vi "GA_Search_Main_Function.vi"(6 "ReInitialize?":bool, 8 "Stop ButtonRef in":refnum<vi>, 9 "Accuracies Listbox Ref in":refnum<vi>, 10 "Fitness Chart Ref in":refnum<vi>, 11 "GA Metaparameters in":T1={"Training Data Path"=path "", "Test Data Path"=path "", "True Labels for Test Trials"=path "", "ClassifierType"=enum."Multilayer perceptron", "SVM Options"={"Kernel"=enum."Linear", "Degree"=0, "Gamma"=0.0, "Coefficient"=0.0, "Sigma"=0.0, "Cache(MB)"=0.0}, "GA Parameters"={"Population size"=0, "Generations no."=0, "Crossover probabality"=0.0, "Mutation mode"=enum."one-point, fixed rate", "Creep mutation"=FALSE, "Mutation rate"=0.0, "Min mutation rate"=0.0, "Max mutation rate"=0.0, "Relative fitness differential"=0.0, "Reproduction plan"=enum."Full generational replacement", "Elitism"=FALSE, "FeaturesPerChannel"=0}, "Use equal number of trials?"=FALSE, "Classifier Metaparameter"=5.0, "ClassifierQualityMeasure"=enum."Accuracy"} {"Classifier Metaparameter" min=0.0 max=100.0 step=0.1 format="%#_2g"; "GA Parameters"."Relative fitness differential" min=0.0 max=1.0; "GA Parameters"."Max mutation rate" min=0.0 max=1.0; "GA Parameters"."Min mutation rate" min=0.0 max=1.0; "GA Parameters"."Mutation rate" min=0.0 max=1.0; "GA Parameters"."Crossover probabality" min=0.0 max=1.0; "GA Parameters"."Generations no." min=1; "GA Parameters"."Population size" min=1}) -> (0 "Accuracies out (double)":dbl[](array[numeric]), 3 "Accuracies out (string)":string[](array[string]))   [LabVIEW 2016, in "GA.lvlib"]
uses:
  _vlib/GA_tSolution progress.ctl
  _vlib/GA_tPopulation.ctl
  _vlib/GA_metaParameters.ctl
  4. Accuracy Assessment for EEG Classification/_vlib/CU_ClassifierTypes.ctl
  <vilib>/vision/Classification.llb/IMAQ SVM Kernel Options.ctl
  _vlib/GA_tParameters.ctl
  4. Accuracy Assessment for EEG Classification/_vlib/CU_ClassifierQualityMeasure.ctl
  _vlib/GA_ApplicationState.ctl
  4. Accuracy Assessment for EEG Classification/_vlib/ClassifierClass.lvclass
  4. Accuracy Assessment for EEG Classification/_vlib/ClassifierClass.lvclass/ClassifierClass.ctl
  _vlib/GA_tFitness Function.ctl
  _vlib/GA.lvlib
  4. Accuracy Assessment for EEG Classification/Classifier.lvlib
panel:
  out "Number of classes":i32 caption="Число классов"
  out "Feature Vector Length":i32 caption="Длина вектора признаков"
  out "Number of True Labels":i32 caption="Число меток классов"
  out "Number of Test Trials":i32 caption="Число тестовых проб"
  out "Number of Training Trials":i32 caption="Число обучающих проб"
  out "Number of trials of each class":i32[](array[numeric]) caption="Число проб каждого класса"
  out "Population Notifier":refnum<notifier>
  out "Solution Notifier":refnum<notifier>
  out "Application State":string caption="Состояние"
  # "This VI is a part of BCI Design library, http://www.ru-bci.org \nCopyright © 2020, Sotnikov Peter, All rights reserved. License: GNU GPLv3"
  # "Поколение"
  # "Точность\nна тестовой\nвыборке"
  # "Размерность\nвектора\nпризнаков"
  # "Точность\nна обучающей\nвыборке"
  # "Точность\nна контрол. \nвыборке"
  # "Результаты чтения данных"
  # "Размер популяции"
  # "Число поколений"
  # "Вероятность скрещивания (кроссовера)"
  # "Тип мутации"
  # "Вероятность мутации"
  # "Минимальная вероятность мутации"
  # "Максимальная вероятность мутации"
  # "Способ включения потомков в популяцию"
  # "Использовать элитизм?"
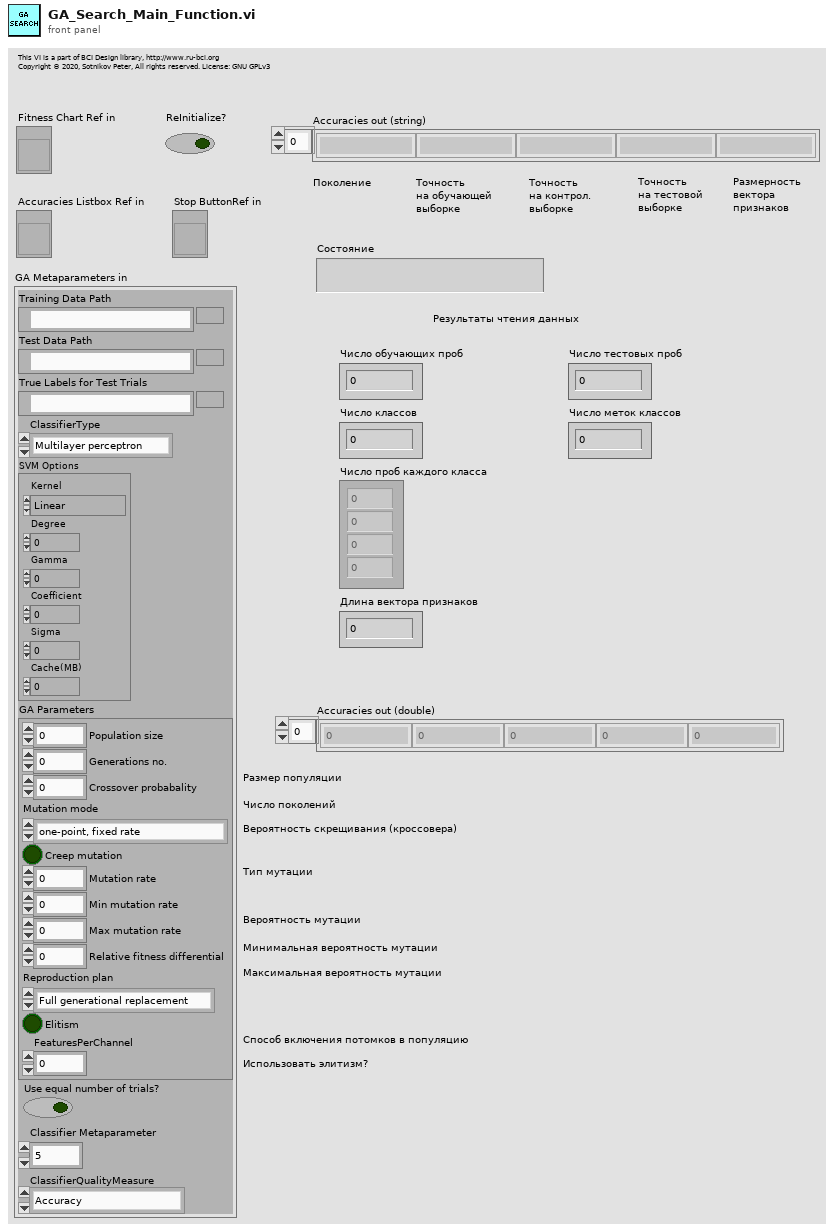
[diagram p1: front panel]
types:
  T1 = typedef "GA.lvlib/GA_metaParameters.ctl" = cluster{"Training Data Path":path, "Test Data Path":path, "True Labels for Test Trials":path, "ClassifierType":T2, "SVM Options":T3, "GA Parameters":T4, "Use equal number of trials?":bool, "Classifier Metaparameter":dbl, "ClassifierQualityMeasure":T5}
  T2 = typedef "Classifier.lvlib/CU_ClassifierTypes.ctl" = enum16{"Multilayer perceptron", "k NN Classifier", "SVM Committee", "Mahalanobis distance", "SVM Classifier"}
  T3 = typedef "IMAQ SVM Kernel Options.ctl" = cluster{"Kernel":enum32{"Linear", "Polynomial", "Gaussian", "RBF"}, "Degree":i32, "Gamma":dbl, "Coefficient":dbl, "Sigma":dbl, "Cache(MB)":dbl}
  T4 = typedef "GA.lvlib/GA_tParameters.ctl" = cluster{"Population size":i32, "Generations no.":i32, "Crossover probabality":dbl, "Mutation mode":enum16{"one-point, fixed rate", "one-point, fitness-adjustable rate", "one-point, distance-adjustable rate"}, "Creep mutation":bool, "Mutation rate":dbl, "Min mutation rate":dbl, "Max mutation rate":dbl, "Relative fitness differential":dbl, "Reproduction plan":enum16{"Full generational replacement", "Steady-state-replace-random", "Steady-state-replace-worst"}, "Elitism":bool, "FeaturesPerChannel":i32}
  T5 = typedef "Classifier.lvlib/CU_ClassifierQualityMeasure.ctl" = enum16{"Accuracy", "Cohen's kappa"}
  T6 = typedef "GA.lvlib/GA_ApplicationState.ctl" = enum16{"Start", "Read Data", "GA in Progress", "Stop"}
  T7 = typedef "GA.lvlib/GA_tFitness Function.ctl" = refnum<vi>
  T8 = cluster{"Training Data Path":path, "Test Data Path":path, "True Labels for Test Trials":path}
  T9 = cluster{"Number of Classes":i32, "NumberOfTrials":i32, "NumberOfTrials":i32, "Number of labels":i32}
  T10 = typedef "GA.lvlib/GA_tSolution progress.ctl" = cluster{"Solution":i8[], "Fitness":dbl, "Mutation rate":dbl, "Generation":i32}
  T11 = typedef "GA.lvlib/GA_tPopulation.ctl" = cluster{"Population":i8[][], "Fitnesses":dbl[], "Sorted indices":i32[], "Ranks":i32[]}
  T12 = cluster{"Fitness Chart Ref in":refnum<vi>, "Accuracies Listbox Ref in":refnum<vi>}
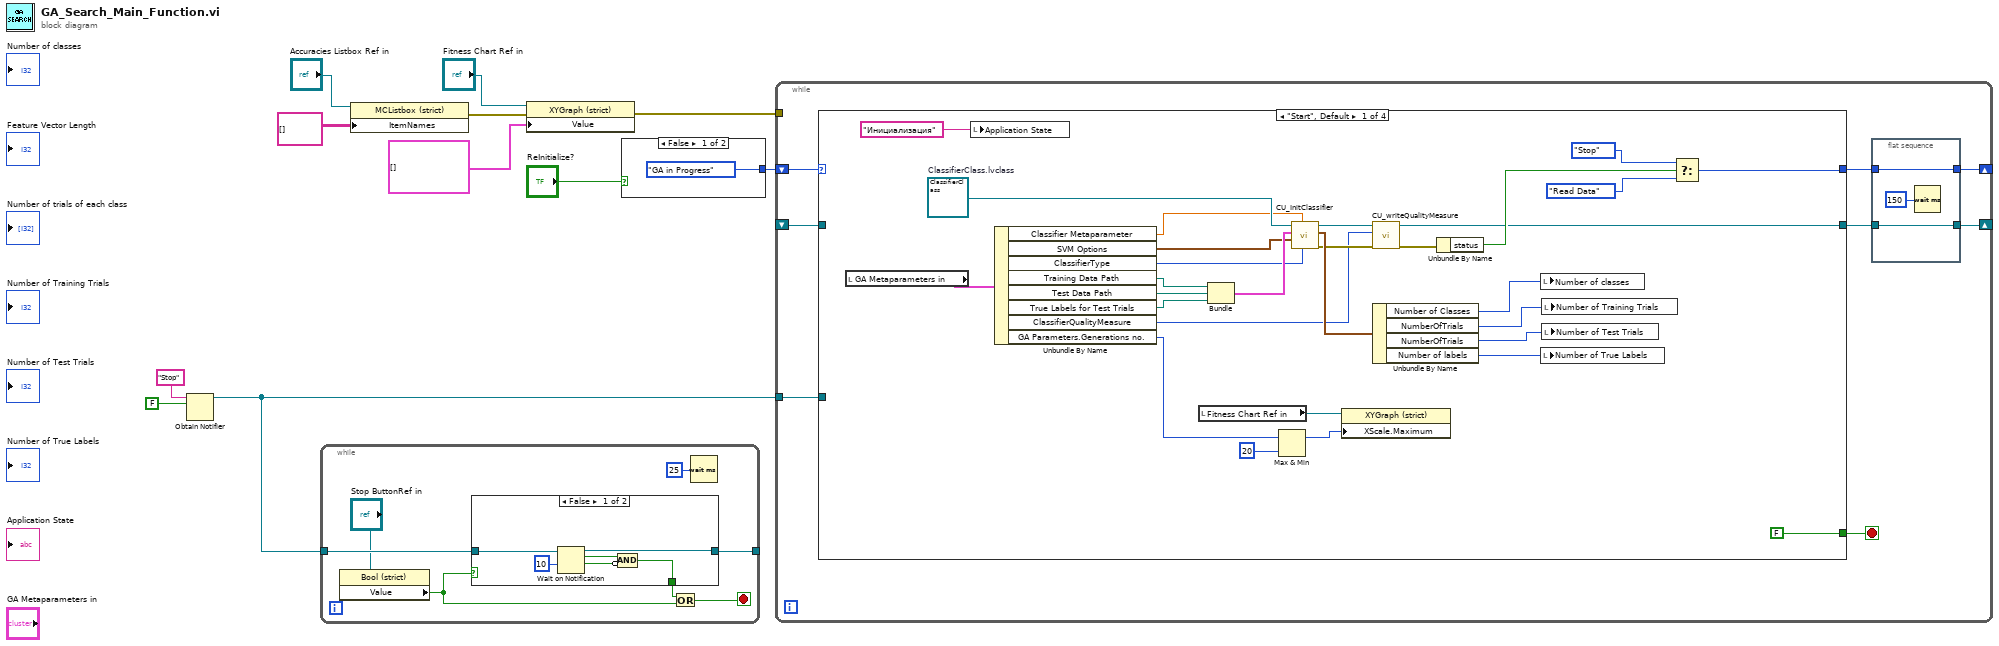
[diagram p0: block diagram]
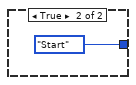
[diagram p2: hidden frame]
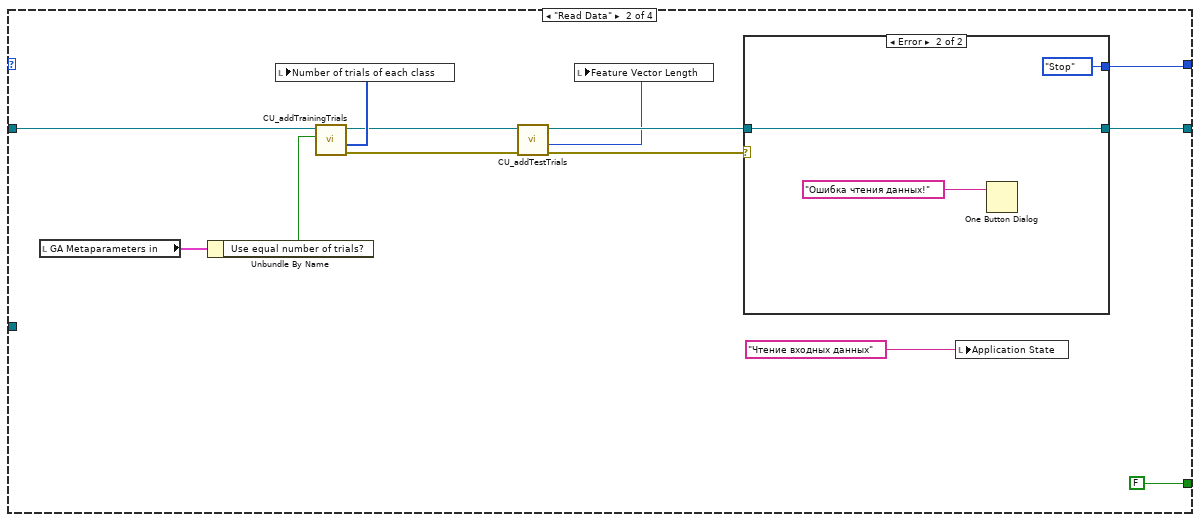
[diagram p3: hidden frame]
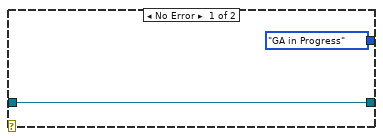
[diagram p4: hidden frame]
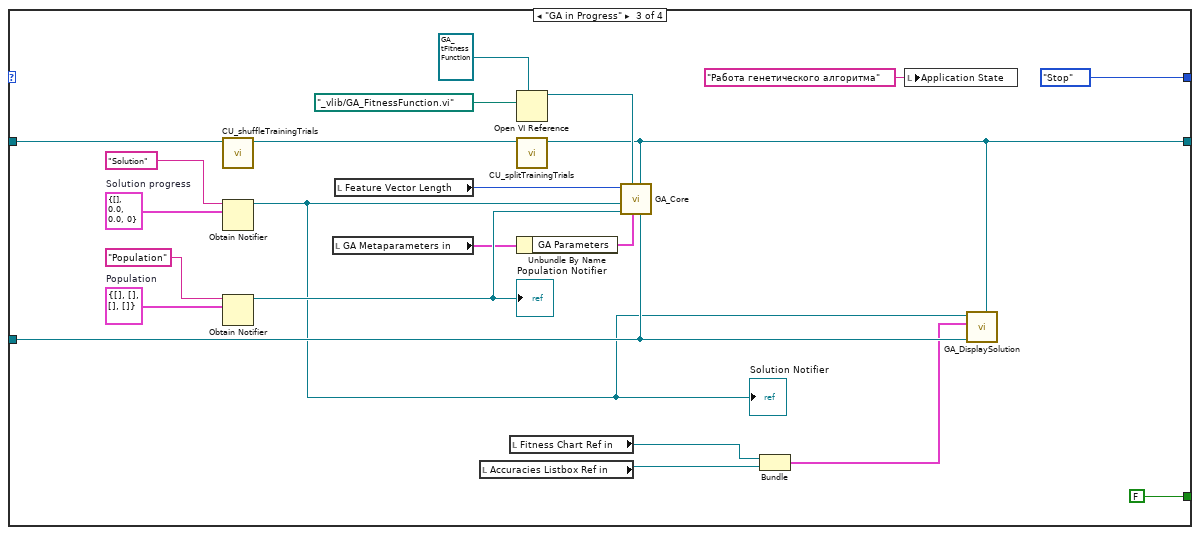
[diagram p5: hidden frame]
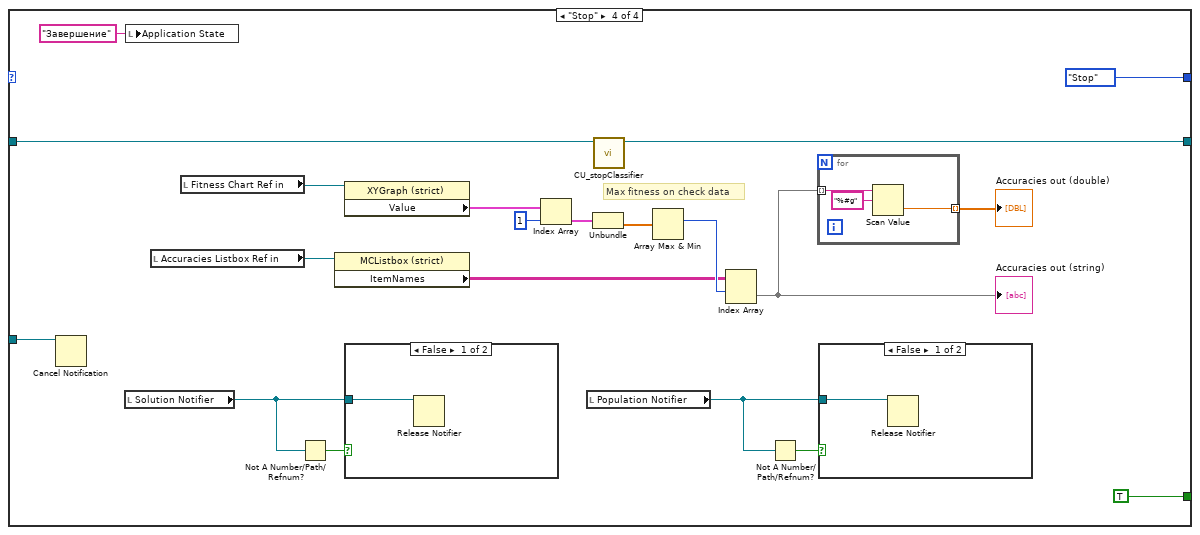
[diagram p6: hidden frame]
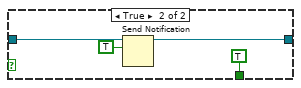
[diagram p9: hidden frame]
diagram:
  n1 = Obtain Notifier(name (unnamed)="Stop", notification data type=FALSE) -> (notifier out=w8:refnum<notifier>)  [unwired: 2 in, 2 out]
  n2 = while {
    tunnel: w8 -> [w17]
    tunnel: [w16] -> _
    stop <- w12 stop-if-true
    n3 = property class="Bool (strict)"(reference="Stop ButtonRef in") -> ("Value"=w13:bool)  [unwired: 1 in, 2 out]
    n4 = case shown="False" w13 {
      tunnel: w17 -> [w21 w28]
      tunnel: [w20 w26] -> w16
      tunnel: [w19 TRUE] -> w14
      frame False {
        n5 = Wait on Notification(notifier=w21, timeout in ms (-1)=10) -> (notifier out=w20:refnum<notifier>, notification=w23:bool, timed out?=w24:bool)  [unwired: 2 in, 1 out]
        n6 = Compound Arithmetic op=AND(w23, invert w24) -> (w19:bool)
      }
      frame True {
        n7 = Send Notification(notification=TRUE, notifier=w28) -> (notifier out=w26:refnum<notifier>)  [unwired: 1 in, 1 out]
      }
    }
    n8 = Or(x=w14, y=w13) -> (x .or. y?=w12:bool)
    n9 = Wait (ms)(milliseconds to wait=u32 25) -> ()  [unwired: 1 out]
  }
  n10 = property class="MCListbox (strict)"(reference="Accuracies Listbox Ref in", "ItemNames"=string[][] [] ("Item Names")) -> (error out=w4:errorcluster)  [unwired: 1 in, 1 out]
  n11 = property class="XYGraph (strict)"(reference="Fitness Chart Ref in", error in=w4, "Value"=cluster{i32[], dbl[]}[] [] ("Fitness Chart")) -> (error out=w2:errorcluster)  [unwired: 1 out]
  n12 = case shown="False" "ReInitialize?" {
    tunnel: [GA_ApplicationState."GA in Progress" ("ApplicationState") GA_ApplicationState."Start" ("ApplicationState")] -> w11
    frame False {
    }
    frame True {
    }
  }
  n13 = while {
    shift-right: [w35] -> _
    shift-left: w11 -> [w31]
    shift-right: [w32] -> _
    shift-left: _ -> [w38]
    tunnel: w8 -> [w36]
    tunnel: w2 -> [_]
    stop <- w37 stop-if-true
    n14 = case shown="\"Start\", Default" w31 {
      tunnel: w38 -> [_ w78 w91 w128]
      tunnel: [FALSE ("Stop Button") FALSE ("Stop Button") FALSE ("Stop Button") TRUE ("Stop Button")] -> w37
      tunnel: [w59 w82 GA_ApplicationState."Stop" ("ApplicationState") GA_ApplicationState."Stop" ("ApplicationState")] -> w34
      tunnel: [w42 w80 w89 w127] -> w33
      tunnel: w36 -> [_ _ w109 w113]
      frame "Start", Default {
        w52 = refnum<class "ClassifierClass.lvclass"> refnum  # ClassifierClass.lvclass
        n15 = local read "GA Metaparameters in"() -> (w58:T1)
        n16 = local write "Application State"("Инициализация" ("Application State")) -> ()
        n17 = Unbundle By Name(w58) -> ("Classifier Metaparameter"=w48:dbl, "SVM Options"=w53:T3, "ClassifierType"=w57:T2, "Training Data Path"=w56:path, "Test Data Path"=w55:path, "True Labels for Test Trials"=w54:path, "ClassifierQualityMeasure"=w43:T5, "GA Parameters.Generations no."=w47:i32)
        n18 = local read "Fitness Chart Ref in"() -> (w51:refnum<vi>)
        n19 = Bundle("Training Data Path"=w56, "Test Data Path"=w55, "True Labels for Test Trials"=w54) -> (w68:T8)  [unwired: 1 in]
        n20 = Max & Min(x=w47, y=20) -> (max(x,y)=w49:i32)  [unwired: 1 out]
        n21 = call "CU_InitClassifier.vi"("ClassifierType"=w57, "Classifier Metaparameter"=w48, "Kernel Options"=w53, "Paths"=w68, "ClassifierClass in"=w52) -> ("error out"=w46:errorcluster, "Number of Trials"=w67:T9, "ClassifierClass out"=w45:refnum<class "ClassifierClass.lvclass">)  [unwired: 4 in]
        n22 = property class="XYGraph (strict)"(reference=w51, "XScale.Maximum"=w49) -> ()  [unwired: 1 in, 2 out]
        n23 = call "CU_writeQualityMeasure.vi"("error in (no error)"=w46, "ClassifierQualityMeasure in"=w43, "ClassifierClass in"=w45) -> ("error out"=w44:errorcluster, "ClassifierClass out"=w42:refnum<class "ClassifierClass.lvclass">)  [unwired: 7 in]
        n24 = Unbundle By Name(w67) -> ("Number of Classes"=w60:i32, "NumberOfTrials"=w66:i32, "NumberOfTrials"=w65:i32, "Number of labels"=w61:i32)
        n25 = Unbundle By Name(w44) -> ("status"=w64:bool)
        n26 = local write "Number of classes"(w60) -> ()
        n27 = local write "Number of True Labels"(w61) -> ()
        n28 = local write "Number of Training Trials"(w66) -> ()
        n29 = local write "Number of Test Trials"(w65) -> ()
        n30 = Select(t=GA_ApplicationState."Stop" ("ApplicationState"), s=w64, f=GA_ApplicationState."Read Data" ("ApplicationState")) -> (s? t:f=w59:T6)
      }
      frame "Read Data" {
        n31 = local read "GA Metaparameters in"() -> (w74:T1)
        n32 = Unbundle By Name(w74) -> ("Use equal number of trials?"=w73:bool)
        n33 = call "CU_addTrainingTrials.vi"("Use equal number of trials?"=w73, "ClassifierClass in"=w78) -> ("error out"=w71:errorcluster, "Num of Trials of each Class"=w75:i32[], "ClassifierClass out"=w72:refnum<class "ClassifierClass.lvclass">)  [unwired: 6 in, 1 out]
        n34 = local write "Number of trials of each class"(w75) -> ()
        n35 = call "CU_addTestTrials.vi"("error in (no error)"=w71, "ClassifierClass in"=w72) -> ("error out"=w76:errorcluster, "FeatureVectorLength"=w77:i32, "ClassifierClass out"=w81:refnum<class "ClassifierClass.lvclass">)  [unwired: 6 in, 1 out]
        n36 = local write "Feature Vector Length"(w77) -> ()
        n37 = case shown="Error" w76 {
          tunnel: [GA_ApplicationState."GA in Progress" ("ApplicationState") GA_ApplicationState."Stop" ("ApplicationState")] -> w82
          tunnel: w81 -> [w84 w87]
          tunnel: [w84 w87] -> w80
          frame No Error {
          }
          frame Error {
            n38 = One Button Dialog(message="Ошибка чтения данных!") -> ()  [unwired: 1 in, 1 out]
          }
        }
        n39 = local write "Application State"("Чтение входных данных" ("Application State")) -> ()
      }
      frame "GA in Progress" {
        w105 = T10 {"Solution"=[], "Fitness"=0.0, "Mutation rate"=0.0, "Generation"=0}  # Solution progress
        w107 = T11 {"Population"=[], "Fitnesses"=[], "Sorted indices"=[], "Ranks"=[]}  # Population
        n40 = call-dynamic "CU_shuffleTrainingTrials.vi"("ClassifierClass in"=w91) -> ("ClassifierClass out"=w90:refnum<class "ClassifierClass.lvclass">)  [unwired: 9 in, 1 out]
        n41 = Obtain Notifier(name (unnamed)="Solution", notification data type=w105) -> (notifier out=w99:refnum<notifier>)  [unwired: 2 in, 2 out]
        "Solution Notifier" <- w99
        n42 = Obtain Notifier(name (unnamed)="Population", notification data type=w107) -> (notifier out=w103:refnum<notifier>)  [unwired: 2 in, 2 out]
        "Population Notifier" <- w103
        n43 = local read "GA Metaparameters in"() -> (w95:T1)
        n44 = local read "Feature Vector Length"() -> (w102:i32)
        n45 = local read "Accuracies Listbox Ref in"() -> (w92:refnum<vi>)
        n46 = local read "Fitness Chart Ref in"() -> (w93:refnum<vi>)
        n47 = Open VI Reference(type specifier VI Refnum (for type only)=T7 refnum ("Fitness Function"), vi path=path "_vlib/GA_FitnessFunction.vi") -> (vi reference=w101:T7)  [unwired: 4 in, 1 out]
        n48 = call "CU_splitTrainingTrials.vi"("ClassifierClass in"=w90) -> ("ClassifierClass out"=w89:refnum<class "ClassifierClass.lvclass">)  [unwired: 7 in, 3 out]
        n49 = Unbundle By Name(w95) -> ("GA Parameters"=w94:T4)
        n50 = call "GA_Core.vi"("Stop notifier"=w109, "ClassifierClass.lvclass"=w89, "Parameters"=w94, "Fitness Function"=w101, "Population notifier"=w103, "Solution Progress notifier"=w99, "Phenotype size"=w102) -> ()  [unwired: 2 in, 3 out]
        n51 = Bundle("Fitness Chart Ref in"=w93, "Accuracies Listbox Ref in"=w92) -> (w97:T12)  [unwired: 1 in]
        n52 = local write "Application State"("Работа генетического алгоритма" ("Application State")) -> ()
        n53 = call "GA_DisplaySolution.vi"("ClassifierClass.lvclass"=w89, "Stop Notifier In"=w109, "Controls Refs"=w97, "Solution Notifier In"=w99) -> ()  [unwired: 8 in]
      }
      frame "Stop" {
        # "Max fitness on check data"
        n54 = Cancel Notification(0:w113) -> ()  [unwired: 1 in, 3 out]
        n55 = local read "Solution Notifier"() -> (w122:refnum<notifier>)
        n56 = local write "Application State"("Завершение" ("Application State")) -> ()
        n57 = local read "Accuracies Listbox Ref in"() -> (w115:refnum<vi>)
        n58 = local read "Fitness Chart Ref in"() -> (w117:refnum<vi>)
        n59 = Not A Number/Path/Refnum?(number/path/refnum=w122) -> (NaN/Path/Refnum?=w123:bool)
        n60 = property class="MCListbox (strict)"(reference=w115) -> ("ItemNames"=w114:string[][])  [unwired: 1 in, 2 out]
        n61 = property class="XYGraph (strict)"(reference=w117) -> ("Value"=w116:cluster{i32[], dbl[]}[])  [unwired: 1 in, 2 out]
        n62 = case shown="False" w123 {
          tunnel: w122 -> [w134 _]
          frame False {
            n63 = Release Notifier(notifier=w134) -> ()  [unwired: 2 in, 3 out]
          }
          frame True {
          }
        }
        n64 = Index Array(array=w116, index=1) -> (element=w120:cluster{i32[], dbl[]})
        n65 = local read "Population Notifier"() -> (w124:refnum<notifier>)
        n66 = Unbundle(w120) -> (w119:dbl[])  [unwired: 1 out]
        n67 = call "CU_stopClassifier.vi"("ClassifierClass in"=w128) -> ("ClassifierClass out"=w127:refnum<class "ClassifierClass.lvclass">)  [unwired: 9 in, 1 out]
        n68 = Array Max & Min(array=w119) -> (max index (indices)=w118:i32)  [unwired: 3 out]
        n69 = Index Array(array=w114, index (row)=w118) -> (element=w112:string[])  [unwired: 1 in]
        "Accuracies out (string)" <- w112
        n70 = Not A Number/Path/Refnum?(number/path/refnum=w124) -> (NaN/Path/Refnum?=w125:bool)
        n71 = for {
          tunnel: w112 -> [w133] mode=indexing
          tunnel: [w131] -> w111 mode=indexing
          n72 = Scan Value(string=w133, format string="%#g") -> (value=w131:dbl)  [unwired: 1 in, 1 out]
        }
        "Accuracies out (double)" <- w111
        n73 = case shown="False" w125 {
          tunnel: w124 -> [w135 _]
          frame False {
            n74 = Release Notifier(notifier=w135) -> ()  [unwired: 2 in, 3 out]
          }
          frame True {
          }
        }
      }
    }
    n75 = flat-sequence {
      tunnel: [w40] -> w35
      tunnel: w34 -> [w40]
      tunnel: w33 -> [w39]
      tunnel: [w39] -> w32
      frame #0 {
        n76 = Wait (ms)(milliseconds to wait=u32 150) -> ()  [unwired: 1 out]
      }
    }
  }
